vi "ExPlugin_ROOT.vi"(8 "Error In":errorcluster, 11 "data":string) -> (0 "Error Out":errorcluster, 1 "command":string, 2 "name":string, 3 "Mode out":enum16{"get", "set", "close", "Init", "Check"}(ring))   [LabVIEW 2018]
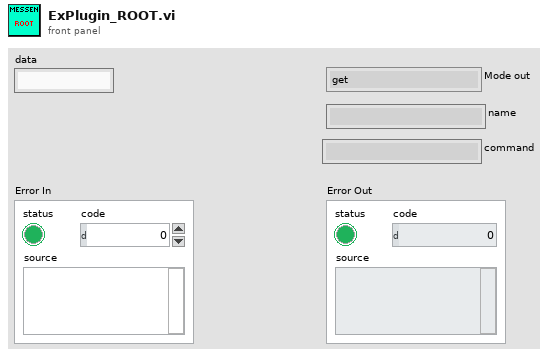
[diagram p1: front panel]
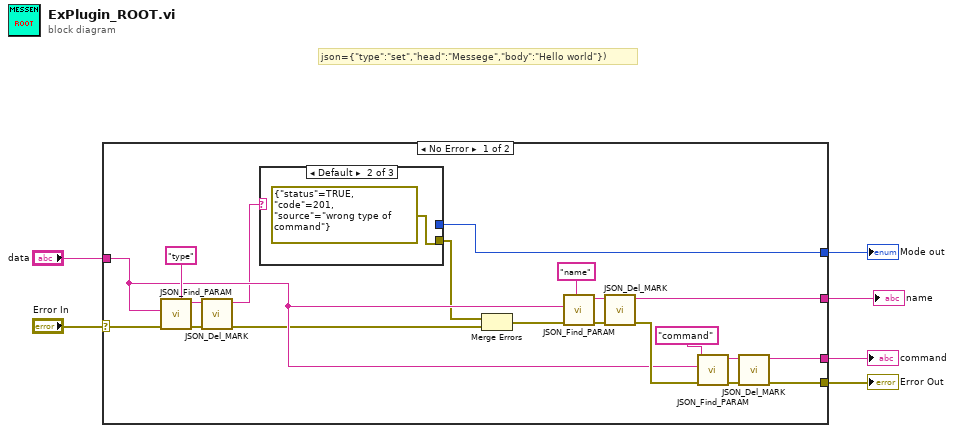
[diagram p0: block diagram]
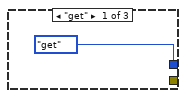
[diagram p2: hidden frame]
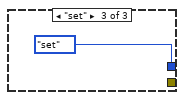
[diagram p3: hidden frame]
diagram:
  # "json={\"type\":\"set\",\"head\":\"Messege\",\"body\":\"Hello world\"})"
  n1 = case shown="No Error" "Error In" {
    selector: "Error In" -> [w14 w30]
    tunnel: "data" -> [w13 _]
    tunnel: [w20 _] -> w5
    tunnel: [w18 w30] -> w3
    tunnel: [w11 _] -> w2
    tunnel: [w7 _] -> w1
    frame No Error {
      n2 = call "JSON_Find_PARAM.vi"("error in (no error)"=w14, "data"=w13, "name"="type") -> ("error out"=w17:errorcluster, "String"=w16:string)  [unwired: 7 in]
      n3 = call "JSON_Del_MARK.vi"("error in (no error)"=w17, "String"=w16) -> ("error out"=w9:errorcluster, "result string"=w12:string)  [unwired: 8 in]
      n4 = case shown="Default" w12 {
        tunnel: [enum16{"get", "set", "close", "Init", "Check"}."get" ("Mode") _ enum16{"get", "set", "close", "Init", "Check"}."set" ("Mode")] -> w11
        tunnel: [_ errorcluster {"status"=TRUE, "code"=201, "source"="wrong type of command"} ("Error") _] -> w10
        frame "get" {
        }
        frame Default {
        }
        frame "set" {
        }
      }
      n5 = Merge Errors(w10, w9) -> (w8:errorcluster)
      n6 = call "JSON_Find_PARAM.vi"("error in (no error)"=w8, "data"=w13, "name"="name") -> ("error out"=w26:errorcluster, "String"=w25:string)  [unwired: 7 in]
      n7 = call "JSON_Del_MARK.vi"("error in (no error)"=w26, "String"=w25) -> ("error out"=w19:errorcluster, "result string"=w7:string)  [unwired: 8 in]
      n8 = call "JSON_Find_PARAM.vi"("error in (no error)"=w19, "data"=w13, "name"="command") -> ("error out"=w23:errorcluster, "String"=w22:string)  [unwired: 7 in]
      n9 = call "JSON_Del_MARK.vi"("error in (no error)"=w23, "String"=w22) -> ("error out"=w18:errorcluster, "result string"=w20:string)  [unwired: 8 in]
    }
    frame Error {
    }
  }
  "command" <- w5
  "Mode out" <- w2
  "Error Out" <- w3
  "name" <- w1
